vi "Excluded units Read.vi"(4 "error in (no error)":errorcluster, 6 "Container State":T2, 7 "Display State In":T1) -> (0 "error out":errorcluster, 2 "Value":enum16{"dB Atten", "dB Vrms", "dB SPL"}[](array[ring]), 3 "Display State Out":T1)   [LabVIEW 2015, in "Level.xctl"]
uses:
  Level.xctl
  <vilib>/_xctls/Container State.ctl
  State.vi
  <vilib>/_xctls/XControlSupport.lvlib
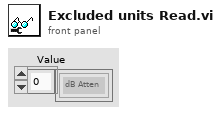
[diagram p1: front panel]
types:
  T1 = typedef "Level.xctl/State.vi" = cluster{"action":string, "excluded":enum16{"dB Atten", "dB Vrms", "dB SPL"}[]}
  T2 = typedef "XControlSupport.lvlib/Container State.ctl" = cluster{"Indicator?":bool, "Run Mode?":bool, " Refnum":refnum<vi>}
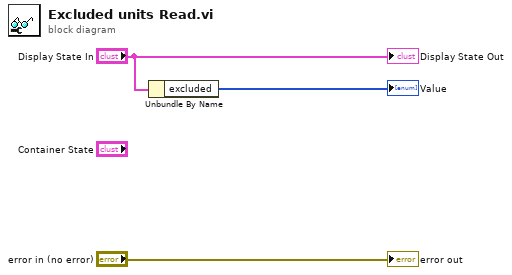
[diagram p0: block diagram]
diagram:
  n1 = Unbundle By Name("Display State In") -> ("excluded"=→"Value":enum16{"dB Atten", "dB Vrms", "dB SPL"}[])
  "error out" <- "error in (no error)"
  "Display State Out" <- "Display State In"
